vi "MovePoint.vi"(3 "Ampitude":dbl, 5 "Freq Y":dbl, 7 "Freq X":dbl, 8 "Amp in":dbl[](array[numeric]), 9 "Y in":u32[](array[numeric]), 10 "X in":u32[](array[numeric]), 11 "Index":i32) -> (0 "Amp out":dbl[](array[numeric]), 1 "Y out":u32[](array[numeric]), 2 "X out":u32[](array[numeric]))   [LabVIEW 2017, in "AODControl.lvlib"]
uses:
  AODControl.lvlib
  CodifyFrequency(Single).vi
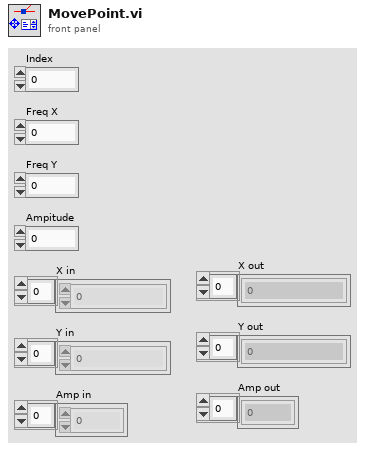
[diagram p1: front panel]
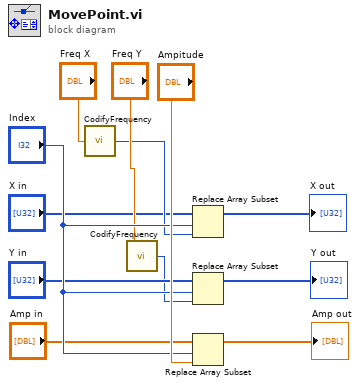
[diagram p0: block diagram]
diagram:
  n1 = call-poly "CodifyFrequency.vi"("Frequency In"="Freq X") -> ("32bit integer"=w3:u32)
  n2 = call-poly "CodifyFrequency.vi"("Frequency In"="Freq Y") -> ("32bit integer"=w4:u32)
  n3 = Replace Array Subset(array="X in", new element=w3, index="Index") -> (→"X out":u32[])
  n4 = Replace Array Subset(array="Y in", new element=w4, index="Index") -> (→"Y out":u32[])
  n5 = Replace Array Subset(array="Amp in", new element="Ampitude", index="Index") -> (→"Amp out":dbl[])
